vi "GET HEWH Faults.vi"(11 "Data":string) -> (3 "Faults":T1 caption="Faul Count")   [LabVIEW 2016]
uses:
  Type Definitions/GEA3 HEWH Faults.ctl
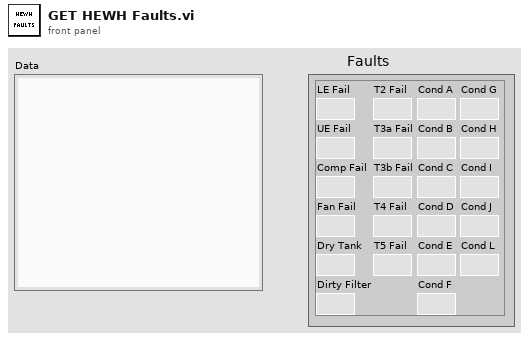
[diagram p1: front panel]
types:
  T1 = typedef "GEA3 HEWH Faults.ctl" = cluster{"LE Fail":u32, "UE Fail":u32, "Comp Fail":u32, "T2 Fail":u32, "T3a Fail":u32, "T3b Fail":u32, "T4 Fail":u32, "T5 Fail":u32, "Cond A":u32, "Cond B":u32, "Cond C":u32, "Cond D":u32, "Cond E":u32, "Cond F":u32, "Cond G":u32, "Cond H":u32, "Cond I":u32, "Cond J":u32, "Cond L":u32, "Fan Fail":u32, "Dirty Filter":u32, "Dry Tank":u32}
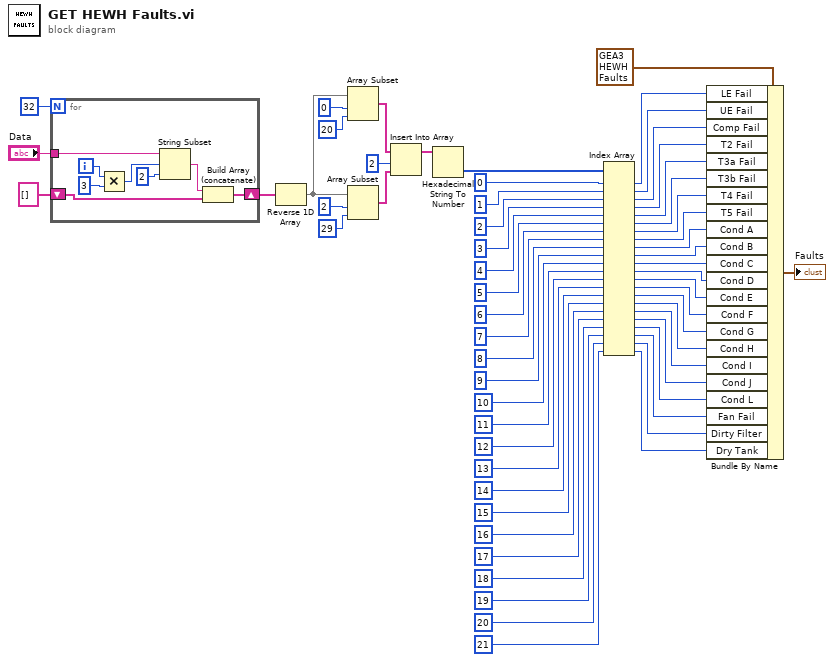
[diagram p0: block diagram]
diagram:
  n1 = for {
    N: 32 -> [_]
    shift-right: [w63] -> w59
    shift-left: string[] [] -> [w62]
    tunnel: "Data" -> [w61]
    i -> [w66]
    n2 = Multiply(x=w66, y=3) -> (x*y=w67:i32)
    n3 = String Subset(string=w61, offset (0)=w67, length (rest)=2 ("length (rest)")) -> (substring=w64:string)
    n4 = Build Array (concatenate)(w64, w62) -> (w63:string[])
  }
  n5 = Reverse 1D Array(array=w59) -> (reversed array=w50:string[])
  n6 = Array Subset(array=w50, index=0, length=20) -> (w52:string[])
  n7 = Array Subset(array=w50, index=2, length=29) -> (w53:string[])
  n8 = Insert Into Array(array=w52, index=2, new element=w53) -> (w54:string[])
  n9 = Hexadecimal String To Number(string=w54) -> (number=w45:u32[])  [unwired: 2 in, 1 out]
  n10 = Index Array(array=w45, index #1=0 ("index"), index #2=1 ("index"), index #3=2 ("index"), index #4=3 ("index"), index #5=4 ("index"), index #6=5 ("index"), index #7=6 ("index"), index #8=7 ("index"), index #9=8 ("index"), index #10=9 ("index"), index #11=10 ("index"), index #12=11 ("index"), index #13=12 ("index"), index #14=13 ("index"), index #15=14 ("index"), index #16=15 ("index"), index #17=16 ("index"), index #18=17 ("index"), index #19=18 ("index"), index #20=19 ("index"), index #21=20 ("index"), index #22=21 ("index")) -> (element #1=w44:u32, element #2=w43:u32, element #3=w42:u32, element #4=w41:u32, element #5=w40:u32, element #6=w39:u32, element #7=w38:u32, element #8=w37:u32, element #9=w36:u32, element #10=w35:u32, element #11=w34:u32, element #12=w33:u32, element #13=w32:u32, element #14=w31:u32, element #15=w30:u32, element #16=w29:u32, element #17=w28:u32, element #18=w27:u32, element #19=w26:u32, element #20=w25:u32, element #21=w24:u32, element #22=w23:u32)
  n11 = Bundle By Name(cluster=T1 {"LE Fail"=0, "UE Fail"=0, "Comp Fail"=0, "T2 Fail"=0, "T3a Fail"=0, "T3b Fail"=0, "T4 Fail"=0, "T5 Fail"=0, "Cond A"=0, "Cond B"=0, "Cond C"=0, "Cond D"=0, "Cond E"=0, "Cond F"=0, "Cond G"=0, "Cond H"=0, "Cond I"=0, "Cond J"=0, "Cond L"=0, "Fan Fail"=0, "Dirty Filter"=0, "Dry Tank"=0} ("Fault Count"), "LE Fail"=w44, "UE Fail"=w43, "Comp Fail"=w42, "T2 Fail"=w41, "T3a Fail"=w40, "T3b Fail"=w39, "T4 Fail"=w38, "T5 Fail"=w37, "Cond A"=w36, "Cond B"=w35, "Cond C"=w34, "Cond D"=w33, "Cond E"=w32, "Cond F"=w31, "Cond G"=w30, "Cond H"=w29, "Cond I"=w28, "Cond J"=w27, "Cond L"=w26, "Fan Fail"=w25, "Dirty Filter"=w24, "Dry Tank"=w23) -> (→"Faults":T1)
